vi "Hardware-DI-iPhaseLearn.vi"(11 "DSI Reference":refnum<class "DCM-DSI.lvclass">) -> ()   [LabVIEW 2016, in "DSI-RT.lvlib"]
uses:
  DSI-RT.lvlib
  Classes/DCM-DSI/DCM-DSI.lvclass
  <vilib>/Powertrain Controls/Device Drivers/DCM/Rev0/RT/DCM - RT.lvclass/DCM - RT.ctl
  <vilib>/Powertrain Controls/Device Drivers/DCM/Rev0/RT/Read Stop Target.vi
  Classes/DCM-DSI/Read DCM Ref.vi
  Classes/DCM-DSI/Read DI-A Profiles.vi
  Classes/DCM-DSI/Read DI-B Profiles.vi
  Classes/DCM-DSI/Read DI Scope Data.vi
  Classes/DCM-DSI/Read DI Scope dt.vi
  Classes/DCM-DSI/Read DI Scope Ctr.vi
  Classes/DCM-DSI/Write DI-A Profiles.vi
  Classes/DCM-DSI/Write DI-B Profiles.vi
  <vilib>/Powertrain Controls/Device Drivers/DCM/Rev0/RT/DCM - RT.lvclass
  <vilib>/addons/Software Calibration Management/xSCM/CalPoint.xnode
  <vilib>/addons/Software Calibration Management/xSCM/ni_scm.dll
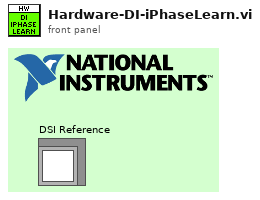
[diagram p1: front panel]
types:
  T1 = enum8{"None", "A1", "A2", "A3", "A4", "A5", "A6", "A7", "A8", "B1", "B2", "B3", "B4", "B5", "B6", "B7", "B8"}
  T2 = cluster{"Mode":enum8{"Off", "Direct", "Calibration", "Triggered Multi-Pulse", "Engine Position Tracking"}, "Digital Input":enum8{"Unused", "User OS", "Diff IO 1", "Diff IO 2", "Diff IO 3", "Diff IO 4", "Diff IO 5", "Diff IO 6", "Diff IO 7", "Diff IO 8", "Aux 1", "Aux 2", "Aux 3", "Aux 4", "Aux 5", "Aux 6", "Aux 7", "Aux 8", "Aux 9", "Aux 10", "Aux 11", "Aux 12", "Aux 13", "Aux 14", "Aux 15", "Aux 16"}, "Default Profile Index":u8, "Cal Freq [Hz]":sgl, "Cal Duration [s]":sgl, "Cal Increment [s]":sgl, "Cal Pulses":u16, "TMP Command Sequence":cluster{"Duration [s]":sgl, "Level":bool, "Run/Stop":bool, "Profile Index":u8}[], "EPT TDC Offset [CAD]":sgl, "EPT Window Start [DBTDC]":sgl, "EPT Window End [DBTDC]":sgl, "EPT Angles":cluster{"Enable":bool, "Timing [DBTDC]":sgl, "Duration [s]":sgl, "Profile Index":u8}[], "EPT Skip Fire":bool, "EPT Skip Index":u8, "EPT Precharge Duration [s]":sgl, "EPT Precharge Profile Index":u8}[]
  T3 = cluster{"Drive":enum8{"Idle", "HV Current Control", "LV Current Control", "Back Boost", "Piezo Charge", "Piezo Discharge"}, "Direction":bool, "Phase Step":enum8{"Duration", "First Peak", "End of Cmd", "Branch", "2-Phase Duration"}, "Duration [s]":sgl, "Current High [A]":sgl, "Current Low [A]":sgl, "Voltage High [V]":sgl, "Voltage Low [V]":sgl, "Change":bool, "Current Control":enum8{"Closed Loop", "Fixed Period", "Fixed On Pulse", "Fixed Off Pulse", "Open Loop", "Profile"}, "Period [s]":sgl, "Pulse Width [s]":sgl, "Profile":u8, "Voltage Control":bool}[][]
  T4 = cluster{"Mode":enum8{"Off", "Direct", "Calibration", "Triggered Multi-Pulse", "Engine Position Tracking"}, "Digital Input":enum8{"Unused", "User OS", "Diff IO 1", "Diff IO 2", "Diff IO 3", "Diff IO 4", "Diff IO 5", "Diff IO 6", "Diff IO 7", "Diff IO 8", "Aux 1", "Aux 2", "Aux 3", "Aux 4", "Aux 5", "Aux 6", "Aux 7", "Aux 8", "Aux 9", "Aux 10", "Aux 11", "Aux 12", "Aux 13", "Aux 14", "Aux 15", "Aux 16"}, "Default Profile Index":u8, "Cal Freq [Hz]":sgl, "Cal Duration [s]":sgl, "Cal Increment [s]":sgl, "Cal Pulses":u16, "TMP Command Sequence":cluster{"Duration [s]":sgl, "Level":bool, "Run/Stop":bool, "Profile Index":u8}[], "EPT TDC Offset [CAD]":sgl, "EPT Window Start [DBTDC]":sgl, "EPT Window End [DBTDC]":sgl, "EPT Angles":cluster{"Enable":bool, "Timing [DBTDC]":sgl, "Duration [s]":sgl, "Profile Index":u8}[], "EPT Skip Fire":bool, "EPT Skip Index":u8, "EPT Precharge Duration [s]":sgl, "EPT Precharge Profile Index":u8}
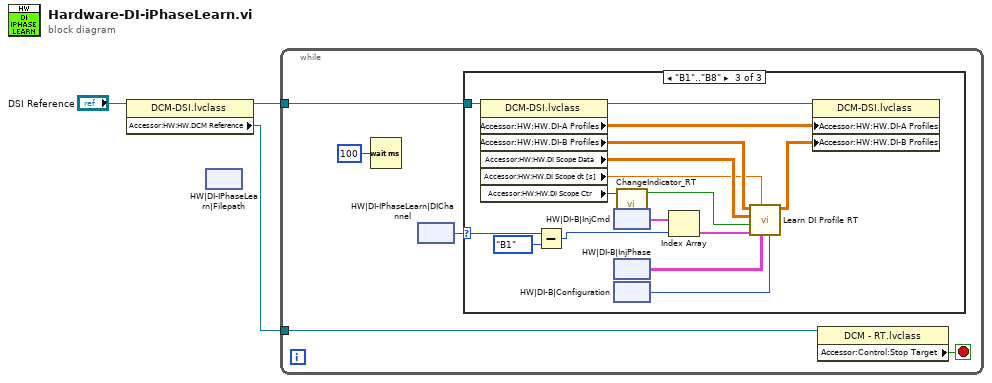
[diagram p0: block diagram]
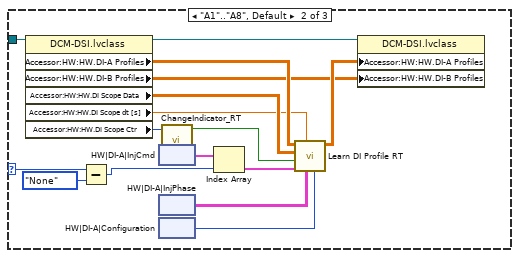
[diagram p3: hidden frame]
diagram:
  n1 = property class="DCM-DSI.lvclass"(reference="DSI Reference") -> (reference out=w2:refnum<class "DCM-DSI.lvclass">, "Accessor:HW:HW.DCM Reference"=w1:refnum<class "DCM - RT.lvclass">)  [unwired: 1 in, 1 out]
  n2 = xnode "HW|DI-IPhaseLearn|Filepath"() -> ()  [unwired: 1 out]
  n3 = while {
    tunnel: w2 -> [w4]
    tunnel: w1 -> [w5]
    stop <- w7 stop-if-true
    n4 = Wait (ms)(milliseconds to wait=u32 100 ("millisecond multiple")) -> ()  [unwired: 1 out]
    n5 = xnode "HW|DI-IPhaseLearn|DIChannel"() -> ("Value"=w8:T1)
    n6 = case shown="\"B1\"..\"B8\"" w8 {
      selector: w8 -> [_ w21 w74]
      tunnel: w4 -> [_ w17 w70]
      frame "None" {
      }
      frame "A1".."A8", Default {
        n7 = property class="DCM-DSI.lvclass"(reference=w17) -> (reference out=w15:refnum<class "DCM-DSI.lvclass">, "Accessor:HW:HW.DI-A Profiles"=w16:sgl[][], "Accessor:HW:HW.DI-B Profiles"=w13:sgl[][], "Accessor:HW:HW.DI Scope Data"=w12:sgl[][], "Accessor:HW:HW.DI Scope dt [s]"=w11:sgl, "Accessor:HW:HW.DI Scope Ctr"=w10:u32)  [unwired: 1 in, 1 out]
        n8 = Subtract(x=w21, y=T1."None" ("Value")) -> (x-y=w19:u8)
        n9 = xnode "HW|DI-A|InjCmd"() -> ("Value"=w24:T2)
        n10 = xnode "HW|DI-A|InjPhase"() -> ("Value"=w23:T3)
        n11 = xnode "HW|DI-A|Configuration"() -> ("Value"=w22:u8)
        n12 = call "ChangeIndicator_RT.vi"("Input"=w10) -> ("Change"=w9:bool)  [unwired: 9 in]
        n13 = Index Array(array=w24, index=w19) -> (element=w18:T4)
        n14 = call "Learn DI Profile RT.vi"("DI Bank Configuration"=w22, "Phase Arrays"=w23, "DI Scope dt [s]"=w11, "Command"=w18, "New Data?"=w9, "DI Scope Data"=w12, "Profiles In"=w16) -> ("Profiles Out"=w14:sgl[][])  [unwired: 4 in]
        n15 = property class="DCM-DSI.lvclass"(reference=w15, "Accessor:HW:HW.DI-A Profiles"=w14, "Accessor:HW:HW.DI-B Profiles"=w13) -> ()  [unwired: 1 in, 2 out]
      }
      frame "B1".."B8" {
        n16 = property class="DCM-DSI.lvclass"(reference=w70) -> (reference out=w69:refnum<class "DCM-DSI.lvclass">, "Accessor:HW:HW.DI-A Profiles"=w66:sgl[][], "Accessor:HW:HW.DI-B Profiles"=w67:sgl[][], "Accessor:HW:HW.DI Scope Data"=w68:sgl[][], "Accessor:HW:HW.DI Scope dt [s]"=w64:sgl, "Accessor:HW:HW.DI Scope Ctr"=w63:u32)  [unwired: 1 in, 1 out]
        n17 = Subtract(x=w74, y=T1."B1" ("Value")) -> (x-y=w72:u8)
        n18 = xnode "HW|DI-B|InjCmd"() -> ("Value"=w77:T2)
        n19 = xnode "HW|DI-B|InjPhase"() -> ("Value"=w76:T3)
        n20 = xnode "HW|DI-B|Configuration"() -> ("Value"=w75:u8)
        n21 = call "ChangeIndicator_RT.vi"("Input"=w63) -> ("Change"=w62:bool)  [unwired: 9 in]
        n22 = Index Array(array=w77, index=w72) -> (element=w71:T4)
        n23 = call "Learn DI Profile RT.vi"("DI Bank Configuration"=w75, "Phase Arrays"=w76, "DI Scope dt [s]"=w64, "Command"=w71, "New Data?"=w62, "DI Scope Data"=w68, "Profiles In"=w67) -> ("Profiles Out"=w65:sgl[][])  [unwired: 4 in]
        n24 = property class="DCM-DSI.lvclass"(reference=w69, "Accessor:HW:HW.DI-A Profiles"=w66, "Accessor:HW:HW.DI-B Profiles"=w65) -> ()  [unwired: 1 in, 2 out]
      }
    }
    n25 = property class="DCM - RT.lvclass"(reference=w5) -> ("Accessor:Control:Stop Target"=w7:bool)  [unwired: 1 in, 2 out]
  }
